vi "Test_PersistToDisk_OverwriteVarLength_ReturnLastValue.vi"(8 "error in (no error)":errorcluster, 11 "TestCase in":refnum<class "TestTransport.lvclass">) -> (0 "error out":errorcluster, 3 "TestCase out":refnum<class "TestTransport.lvclass">)   [LabVIEW 2017, in "TestTransport.lvclass"]
uses:
  TestTransport.lvclass
  Source/Framework/Transport/PersistToDiskTransport/Recovered Value.ctl
  <vilib>/Utility/sysdir.llb/System Directory Type.ctl
  Source/Framework/Transport/PersistToDiskTransport/PersistToDiskTransport.lvclass/PersistToDiskTransport.ctl
  Source/Framework/Transport/PersistToDiskTransport/PersistToDiskTransport.lvclass
panel:
  out "Original Value":T1
  out "Recovered Value":T2
  out "Test Folder Path":path
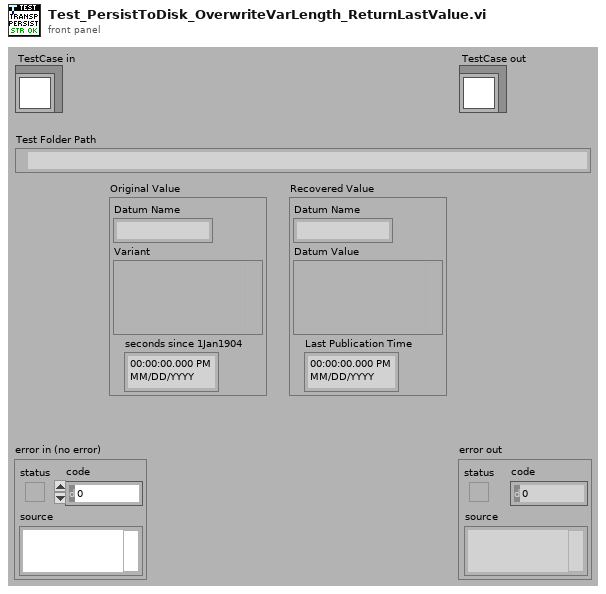
[diagram p1: front panel]
types:
  T1 = cluster{"Datum Name":string, "Variant":variant, "seconds since 1Jan1904":timestamp}
  T2 = typedef "Transport.lvlib/PersistToDiskTransport.lvclass/Recovered Value.ctl" = cluster{"Datum Name":string, "Datum Value":variant, "Last Publication Time":timestamp}
  T3 = typedef "System Directory Type.ctl" = i32
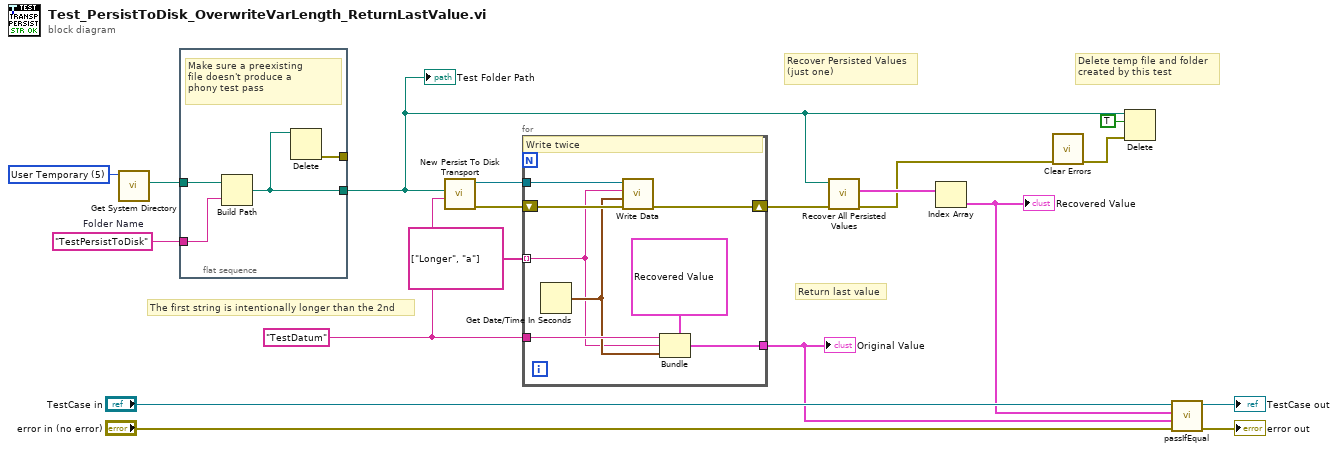
[diagram p0: block diagram]
diagram:
  w9 = "TestDatum" ("Datum Name")
  w12 = "TestPersistToDisk"  # Folder Name
  w14 = T3 5 items=["User Home"=0, "User Desktop"=1, "User Documents"=2, "User Application Data"=3, "User Preferences"=4, "User Temporary"=5, "Public Documents"=6, "Public Application Data"=7, "Public Preferences"=8, "Public Cache"=13, "System Core Libraries"=9, "System Installed Libraries"=10, "Application Files"=11, "Boot Volume Root"=12] ("system directory type")
  # "The first string is intentionally longer than the 2nd"
  # "Return last value"
  # "Delete temp file and folder\ncreated by this test"
  # "Recover Persisted Values\n(just one)"
  n1 = call <vilib>:"Get System Directory.vi"("system directory type"=w14) -> ("system directory"=w13:path)  [unwired: 10 in]
  n2 = flat-sequence {
    tunnel: w13 -> [w22]
    tunnel: [w20] -> w6
    tunnel: [w23] -> _
    tunnel: w12 -> [w21]
    frame #0 {
      # "Make sure a preexisting\nfile doesn't produce a\nphony test pass"
      n3 = Build Path(base path=w22, name or relative path=w21) -> (appended path=w20:path)
      n4 = Delete(path (use dialog)=w20) -> (error out=w23:errorcluster)  [unwired: 4 in, 2 out]
    }
  }
  n5 = call "New Persist To Disk Transport.vi"("Datum Name"=w9, "Folder Path"=w6) -> ("error out"=w15:errorcluster, "PersistToDiskTransport Out"=w16:refnum<class "PersistToDiskTransport.lvclass">)  [unwired: 8 in]
  n6 = for {
    tunnel: w16 -> [w31]
    tunnel: w9 -> [w28]
    tunnel: [w26] -> w8
    shift-right: [w29] -> w11
    shift-left: w15 -> [w30]
    tunnel: string[] ["Longer", "a"] -> [w24] mode=indexing
    # "Write twice"
    n7 = Get Date/Time In Seconds() -> (seconds since 1Jan1904=w27:timestamp)
    n8 = call-dynamic "Write Data.vi"("error in (no error)"=w30, "Publication Time"=w27, "Value"=w24, "PersistToDiskTransport In"=w31) -> ("error out"=w29:errorcluster)  [unwired: 6 in, 1 out]
    n9 = Bundle(cluster=T2 {"Datum Name"="", "Datum Value"=variant, "Last Publication Time"=timestamp(0 s since 1904-01-01)} ("Recovered Value"), "Datum Name"=w28, "Datum Value"=w24, "Last Publication Time"=w27) -> (w26:T2)
  }
  "Original Value" <- w8
  n10 = call "Recover All Persisted Values.vi"("error in (no error)"=w11, "Folder Path"=w6) -> ("error out"=w5:errorcluster, "Recovered Values"=w10:T2[])  [unwired: 8 in]
  n11 = Index Array(array=w10) -> (element=w7:T2)  [unwired: 1 in]
  "Recovered Value" <- w7
  n12 = call <vilib>:"Clear Errors.vi"("error in (no error)"=w5) -> ("error out"=w4:errorcluster)  [unwired: 5 in, 1 out]
  n13 = Delete(path (use dialog)=w6, entire hierarchy (F)=TRUE, error in=w4) -> ()  [unwired: 2 in, 3 out]
  n14 = call-dynamic "passIfEqual.vi"("error in (no error)"="error in (no error)", "y"=w8, "x"=w7, "TestCase in"="TestCase in") -> ("error out"=→"error out":errorcluster, "TestCase out"=→"TestCase out":refnum<class "TestTransport.lvclass">)  [unwired: 6 in]
  "Test Folder Path" <- w6
